vi "Create Tracking Test Waveform.vi"(11 "Model in":refnum<class "Model.lvclass">) -> (2 "Waveform":refnum<class "Waveform.lvclass">, 3 "Model out":refnum<class "Model.lvclass">)   [LabVIEW 2016]
uses:
  Typedefs/WaveformTypes.ctl
  Typedefs/WaveformSettings.ctl
  Model/Waveforms/Waveform Factory/Waveform Factory.lvclass
  Model/Model/Model.lvclass
  Model/Waveforms/Waveform/Waveform.lvclass
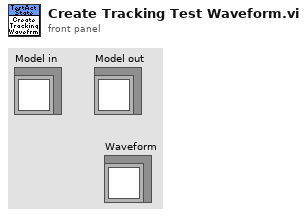
[diagram p1: front panel]
types:
  T1 = typedef "WaveformTypes.ctl" = enum16{"Sine", "Triangle", "Square", "Sawtooth", "Chirp", "Gaussian", "Trapezoid", "Constant"}
  T2 = typedef "WaveformSettings.ctl" = cluster{"Sample Count":u32, "Amplitude":dbl, "Offset":dbl, "Frequency":dbl[unit], "Waveform":T1, "F1":dbl[unit], "F2":dbl[unit], "Duty Cycle":dbl, "ILC Rate":dbl[unit], "Ramp Time":dbl[unit], "Hold Time":dbl[unit], "Settling Time":dbl[unit], "Delay":dbl[unit]}
  T3 = typedef "TrackingTestSettings.ctl" = cluster{"Max Force Error (N)":dbl, "Max Moment (NM)":dbl, "Process Time (s)":dbl, "Sample Time (s)":dbl, "Iterations":i32, "Amplitude (N)":dbl, "Non-Repeating Error":dbl}
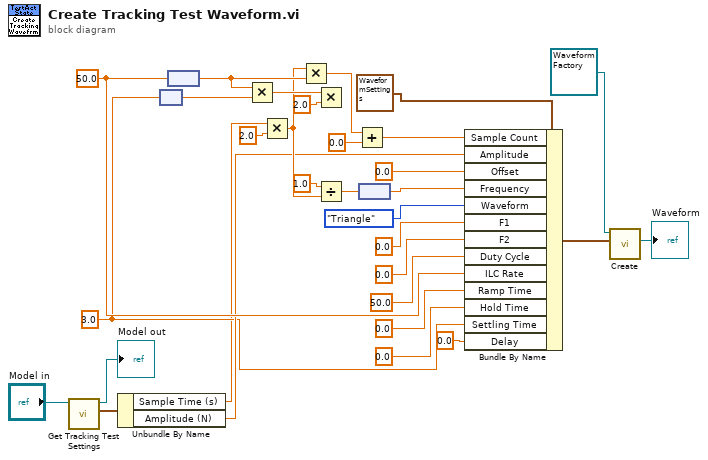
[diagram p0: block diagram]
diagram:
  w5 = dbl[unit] 3.0 ("Settling Time")
  w24 = dbl[unit] 50.0 ("ILC Rate")
  n1 = call "Get Tracking Test Settings.vi"("Model in"="Model in") -> ("Tracking Test Settings"=w12:T3, "Model out"=→"Model out":refnum<class "Model.lvclass">)  [unwired: 9 in]
  n2 = Unbundle By Name(w12) -> ("Sample Time (s)"=w2:dbl, "Amplitude (N)"=w13:dbl)
  n3 = node(w5) -> (w4:dbl)
  n4 = node(w24) -> (w27:dbl)
  n5 = Multiply(x=w27, y=w4) -> (x*y=w28:dbl)
  n6 = Multiply(x=w2, y=2.0) -> (x*y=w25:dbl)
  n7 = Multiply(x=w25, y=w27) -> (x*y=w26:dbl)
  n8 = Multiply(x=w28, y=2.0) -> ()  [unwired: 1 out]
  n9 = Divide(x=1.0, y=w25) -> (x/y=w22:dbl)
  n10 = Add(x=w26, y=0.0) -> (x+y=w30:dbl)
  n11 = node(w22) -> (w23:dbl[unit])
  n12 = Bundle By Name(cluster=T2 {"Sample Count"=0, "Amplitude"=0.0, "Offset"=0.0, "Frequency"=0.0, "Waveform"=enum."Sine", "F1"=0.0, "F2"=0.0, "Duty Cycle"=0.0, "ILC Rate"=0.0, "Ramp Time"=0.0, "Hold Time"=0.0, "Settling Time"=0.0, "Delay"=0.0} ("Waveform Settings"), "Sample Count"=w30, "Amplitude"=w13, "Offset"=0.0, "Frequency"=w23, "Waveform"=WaveformTypes."Triangle", "F1"=dbl[unit] 0.0, "F2"=dbl[unit] 0.0, "Duty Cycle"=50.0, "ILC Rate"=w24, "Ramp Time"=dbl[unit] 0.0, "Hold Time"=dbl[unit] 0.0, "Settling Time"=w5, "Delay"=dbl[unit] 0.0) -> (w7:T2)
  n13 = call-dynamic "Create.vi"("Waveform Settings"=w7, "Waveform Factory in"=refnum<class "Waveform Factory.lvclass"> refnum ("Waveform Factory.lvclass")) -> ("Waveform"=→"Waveform":refnum<class "Waveform.lvclass">)  [unwired: 7 in, 2 out]
